vi "MovePiezo.vi"(0 "MG17 Y in":refnum<k7>, 1 "MG17 X in":refnum<k7>, 2 "MG17 Z in":refnum<k7>, 5 "Y":sgl, 7 "error in X":errorcluster, 9 "error in Z":errorcluster, 11 "error in Y":errorcluster, 12 "Z":sgl, 13 "X":sgl) -> (3 "pfVoltage X":sgl, 4 "MG17 Y out":refnum<k7>, 6 "MG17 Z out":refnum<k7>, 8 "MG17 X out":refnum<k7>, 10 "pfVoltage Z":sgl, 14 "pfVoltage Y":sgl, 15 "error out":errorcluster)   [LabVIEW 2014]
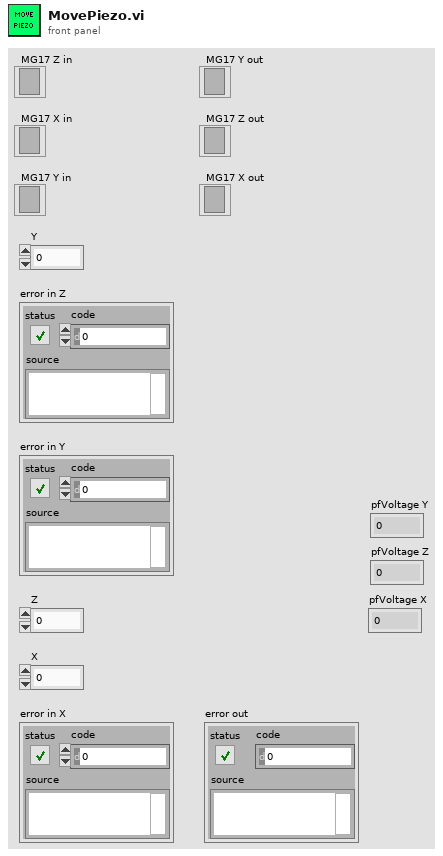
[diagram p1: front panel]
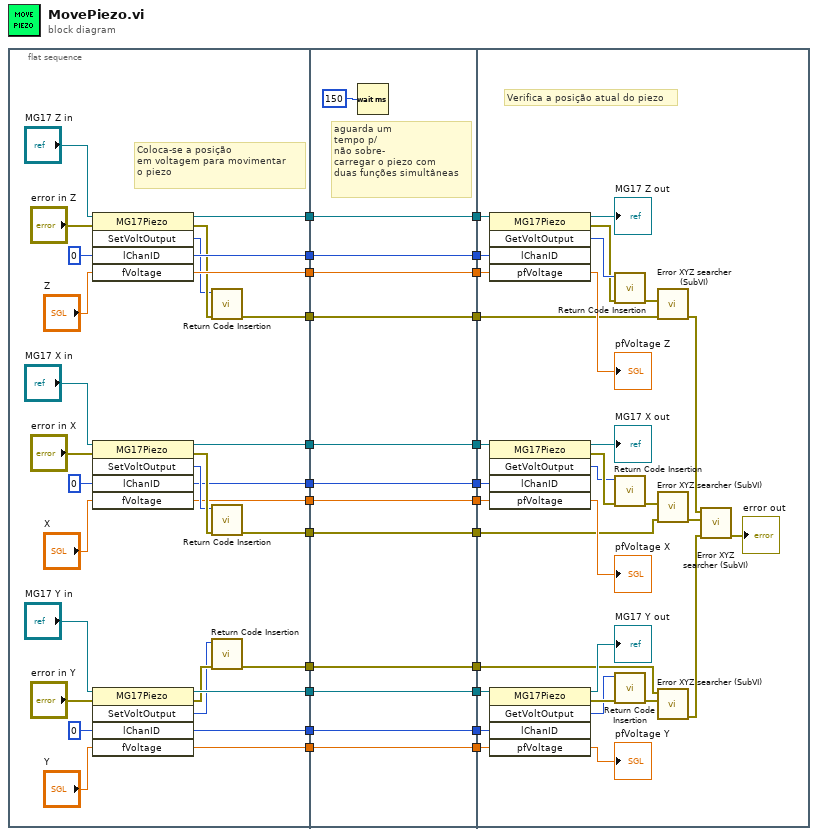
[diagram p0: block diagram]
diagram:
  n1 = flat-sequence {
    tunnel: [w50] -> w24
    tunnel: [w49] -> w22
    tunnel: [w46] -> w20
    tunnel: [w45] -> w18
    tunnel: [w40] -> w15
    tunnel: [w39] -> w14
    tunnel: [w38] -> w12
    tunnel: [w33] -> w9
    tunnel: [w30] -> w7
    tunnel: [w29] -> w5
    tunnel: [w28] -> w3
    tunnel: [w27] -> w1
    tunnel: w24 -> [w67]
    tunnel: [w67] -> w23
    tunnel: w22 -> [w66]
    tunnel: [w66] -> w21
    tunnel: w20 -> [w65]
    tunnel: [w65] -> w19
    tunnel: w18 -> [w64]
    tunnel: [w64] -> w17
    tunnel: [w63] -> w16
    tunnel: w15 -> [w63]
    tunnel: w14 -> [w62]
    tunnel: [w62] -> w13
    tunnel: w12 -> [w61]
    tunnel: [w61] -> w11
    tunnel: [w60] -> w10
    tunnel: w9 -> [w60]
    tunnel: [w59] -> w8
    tunnel: w7 -> [w59]
    tunnel: [w58] -> w6
    tunnel: w5 -> [w58]
    tunnel: [w57] -> w4
    tunnel: w3 -> [w57]
    tunnel: [w56] -> w2
    tunnel: w1 -> [w56]
    tunnel: w23 -> [w93]
    tunnel: w21 -> [w92]
    tunnel: w19 -> [w91]
    tunnel: w17 -> [w90]
    tunnel: w16 -> [w84]
    tunnel: w13 -> [w83]
    tunnel: w11 -> [w82]
    tunnel: w10 -> [w76]
    tunnel: w8 -> [w75]
    tunnel: w6 -> [w74]
    tunnel: w4 -> [w73]
    tunnel: w2 -> [w68]
    frame #0 {
      # "Coloca-se a posição \nem voltagem para movimentar \no piezo"
      n2 = invoke class="MG17Piezo" method="SetVoltOutput"(reference="MG17 Z in", error in="error in Z", "lChanID"=0, "fVoltage"="Z") -> (reference out=w40:refnum<k7>, error out=w26:errorcluster, "SetVoltOutput"=w25:i32, "lChanID"=w38:i32, "fVoltage"=w39:sgl)  [unwired: 1 in]
      n3 = invoke class="MG17Piezo" method="SetVoltOutput"(reference="MG17 X in", error in="error in X", "lChanID"=0, "fVoltage"="X") -> (reference out=w33:refnum<k7>, error out=w32:errorcluster, "SetVoltOutput"=w31:i32, "lChanID"=w29:i32, "fVoltage"=w28:sgl)  [unwired: 1 in]
      n4 = invoke class="MG17Piezo" method="SetVoltOutput"(reference="MG17 Y in", error in="error in Y", "lChanID"=0, "fVoltage"="Y") -> (reference out=w49:refnum<k7>, error out=w48:errorcluster, "SetVoltOutput"=w47:i32, "lChanID"=w50:i32, "fVoltage"=w45:sgl)  [unwired: 1 in]
      n5 = call "Return Code Insertion.vi"("error in (no error)"=w26, "Return Code"=w25) -> ("error out"=w27:errorcluster)  [unwired: 9 in]
      n6 = call "Return Code Insertion.vi"("error in (no error)"=w32, "Return Code"=w31) -> ("error out"=w30:errorcluster)  [unwired: 9 in]
      n7 = call "Return Code Insertion.vi"("error in (no error)"=w48, "Return Code"=w47) -> ("error out"=w46:errorcluster)  [unwired: 9 in]
    }
    frame #1 {
      # "aguarda um\ntempo p/\nnão sobre-\ncarregar o piezo com\nduas funções simultâneas"
      n8 = Wait (ms)(milliseconds to wait=u32 150) -> ()  [unwired: 1 out]
    }
    frame #2 {
      # "Verifica a posição atual do piezo"
      n9 = invoke class="MG17Piezo" method="GetVoltOutput"(reference=w84, "lChanID"=w82, "pfVoltage"=w83) -> (reference out=→"MG17 Z out":refnum<k7>, error out=w87:errorcluster, "GetVoltOutput"=w88:i32, "pfVoltage"=→"pfVoltage Z":sgl)  [unwired: 2 in, 1 out]
      n10 = invoke class="MG17Piezo" method="GetVoltOutput"(reference=w76, "lChanID"=w74, "pfVoltage"=w73) -> (reference out=→"MG17 X out":refnum<k7>, error out=w79:errorcluster, "GetVoltOutput"=w78:i32, "pfVoltage"=→"pfVoltage X":sgl)  [unwired: 2 in, 1 out]
      n11 = invoke class="MG17Piezo" method="GetVoltOutput"(reference=w92, "lChanID"=w93, "pfVoltage"=w90) -> (reference out=→"MG17 Y out":refnum<k7>, error out=w98:errorcluster, "GetVoltOutput"=w97:i32, "pfVoltage"=→"pfVoltage Y":sgl)  [unwired: 2 in, 1 out]
      n12 = call "Return Code Insertion.vi"("error in (no error)"=w87, "Return Code"=w88) -> ("error out"=w89:errorcluster)  [unwired: 9 in]
      n13 = call "Return Code Insertion.vi"("error in (no error)"=w79, "Return Code"=w78) -> ("error out"=w81:errorcluster)  [unwired: 9 in]
      n14 = call "Return Code Insertion.vi"("error in (no error)"=w98, "Return Code"=w97) -> ("error out"=w94:errorcluster)  [unwired: 9 in]
      n15 = call "Error XYZ searcher (SubVI).vi"("error Y"=w68, "error Z"=w89) -> ("error out"=w71:errorcluster)  [unwired: 9 in]
      n16 = call "Error XYZ searcher (SubVI).vi"("error Y"=w75, "error Z"=w81) -> ("error out"=w70:errorcluster)  [unwired: 9 in]
      n17 = call "Error XYZ searcher (SubVI).vi"("error Z"=w94, "error X"=w91) -> ("error out"=w69:errorcluster)  [unwired: 9 in]
      n18 = call "Error XYZ searcher (SubVI).vi"("error Y"=w69, "error Z"=w70, "error X"=w71) -> ("error out"=→"error out":errorcluster)  [unwired: 8 in]
    }
  }
